vi "stC to K.vi"(8 "error in (no error)":errorcluster, 10 "stC (0)":dbl) -> (0 "error out":errorcluster, 2 "K":dbl)   [LabVIEW 2013]
doc: "Konwertuje wartości temperatury między skalą Celcjusza a Kelwina"
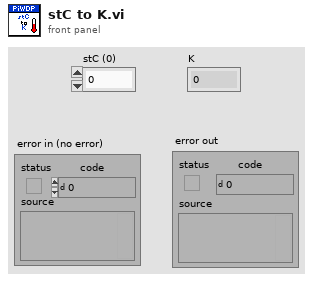
[diagram p1: front panel]
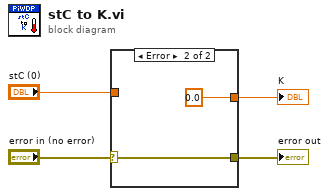
[diagram p0: block diagram]
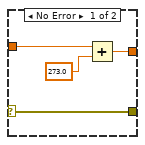
[diagram p2: hidden frame]
diagram:
  n1 = case shown="Error" "error in (no error)" {
    selector: "error in (no error)" -> [w8 w10]
    tunnel: [w8 w10] -> w3
    tunnel: "stC (0)" -> [w7 _]
    tunnel: [w6 0.0] -> w1
    frame No Error {
      n2 = Add(x=w7, y=273.0) -> (x+y=w6:dbl)
    }
    frame Error {
    }
  }
  "error out" <- w3
  "K" <- w1
